vi "calcVoltagesZ.vi"(6 "maxTxVoltageVolt":sgl=128.0 format="%.2f", 7 "Log file":path=path "nologfile", 8 "numMeasVoltage":i8=4, 9 "totalVoltagePt":i8=8, 10 "ceilTxVoltageVolt":sgl=128.0 format="%.2f") -> (2 "Voltages":sgl[](array[numeric])=[128.0, 64.0, 32.0, 16.0] format="%.2f")   [LabVIEW 2016]
doc: "Calculates the list of voltages for voltage-dependent measurements.\nFor i = 0 to numMeasVoltage-1,\nV[i] = maxTxVoltageVolt^((totalVoltagePt-1-i)/(totalVoltagePt-1))\nAny voltages which are greater than ceilTxVoltageVolt are removed and replaced by ceilTxVoltageVolt."
panel:
  out "error out":errorcluster
  in  "error in (no error)":errorcluster
  # "Program constants"
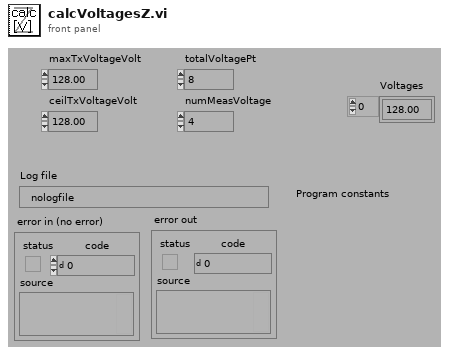
[diagram p1: front panel]
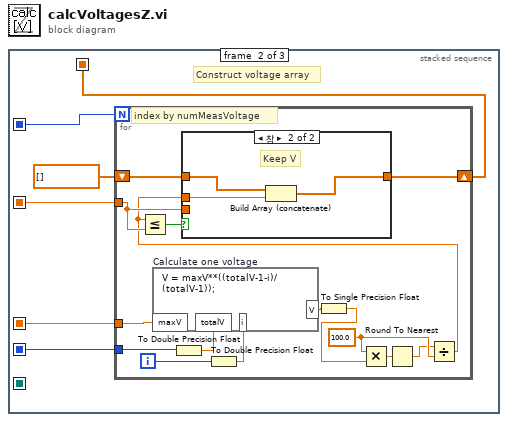
[diagram p0: block diagram]
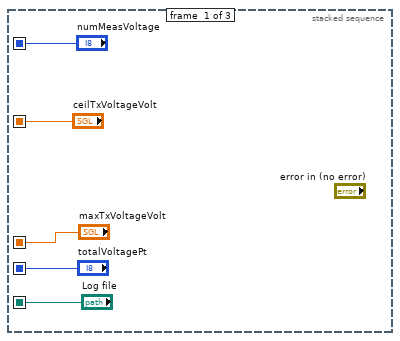
[diagram p2: hidden frame]
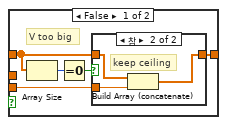
[diagram p3: hidden frame]
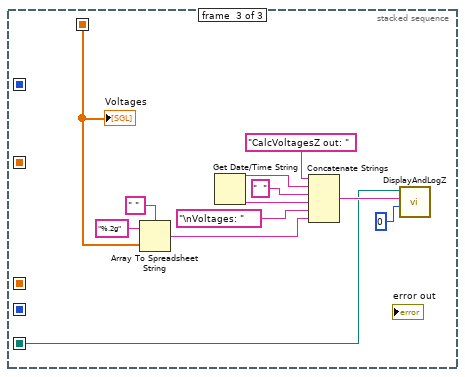
[diagram p5: hidden frame]
diagram:
  n1 = stacked-sequence {
    seq-local: [_ w10 _] -> [_ _ w39]
    seq-local: ["ceilTxVoltageVolt" _ _] -> [_ w9 _]
    seq-local: ["maxTxVoltageVolt" _ _] -> [_ w8 _]
    seq-local: ["totalVoltagePt" _ _] -> [_ w7 _]
    seq-local: ["numMeasVoltage" _ _] -> [_ w6 _]
    seq-local: ["Log file" _ _] -> [_ _ w40]
    frame #0 {
    }
    frame #1 {
      # "Construct voltage array"
      n2 = for {
        N: w6 -> [_]
        shift-right: [w19] -> w10
        shift-left: sgl[] [] ("Voltages") -> [w22]
        tunnel: w8 -> [w23]
        tunnel: w7 -> [w26]
        tunnel: w9 -> [w17]
        i -> [w20]
        w15 = 100.0
        # "index by numMeasVoltage"
        n3 = To Double Precision Float(number=w26) -> (double precision float=w25:dbl)
        n4 = To Double Precision Float(number=w20) -> (double precision float=w24:dbl)
        n5 = formula code="V = maxV**((totalV-1-i)/(totalV-1));" "Calculate one voltage"("totalV"=w25, "maxV"=w23, "i"=w24) -> ("V"=w18:dbl)
        n6 = To Single Precision Float(number=w18) -> (single precision float=w13:sgl)
        n7 = Multiply(x=w15, y=w13) -> (x*y=w16:dbl)
        n8 = Round To Nearest(number=w16) -> (nearest integer value=w14:dbl)
        n9 = Divide(x=w14, y=w15) -> (x/y=w12:dbl)
        n10 = Less Or Equal?(x=w12, y=w17) -> (x <= y?=w21:bool)
        n11 = case shown="참" w21 {
          tunnel: [w29 w36] -> w19
          tunnel: w22 -> [w28 w38]
          tunnel: w12 -> [_ w37]
          tunnel: w17 -> [w27 _]
          frame False {
            # "V too big"
            n12 = Array Size(array=w28) -> (size(s)=w31:i32)
            n13 = Equal To 0?(x=w31) -> (x = 0?=w30:bool)
            n14 = case shown="참" w30 {
              tunnel: [w32 w33] -> w29
              tunnel: w28 -> [w32 w35]
              tunnel: w27 -> [_ w34]
              frame False {
                # "ceiling already\nin array"
              }
              frame True {
                # "keep ceiling"
                n15 = Build Array (concatenate)(w35, w34) -> (w33:dbl[])
              }
            }
          }
          frame True {
            # "Keep V"
            n16 = Build Array (concatenate)(w38, w37) -> (w36:dbl[])
          }
        }
      }
    }
    frame #2 {
      n17 = Array To Spreadsheet String(delimiter (Tab)=" ", array=w39, 3:"%.2g" ("format string")) -> (spreadsheet string=w50:string)
      n18 = Get Date/Time String() -> (date string=w43:string, time string=w45:string)  [unwired: 3 in]
      n19 = Concatenate Strings("CalcVoltagesZ out: " ("Substring"), w43, "  ", w45, "\nVoltages: " ("Substring"), w50) -> (w47:string)
      n20 = call "DisplayAndLogZ.vi"("Log file"=w40, "message"=w47, "action (0: log+display)"=u16 0) -> ()  [unwired: 5 in, 1 out]
      "Voltages" <- w39
    }
  }
